vi "RMGetResults.vi"(8 "error in (no error)":errorcluster, 9 "startFrame (0)":i32, 10 "numFrames":i32, 11 "ResultManager":T4) -> (0 "error out":errorcluster, 2 "results":T1[][](array[typedef]), 3 "ResultManager (out)":T4)   [LabVIEW 2011]
uses:
  QTrkDLL.vi
  XYZf.ctl
  QTrkLocalizationJob.ctl
  QTrkLocalizationResult.ctl
  ResultManagerInstance.ctl
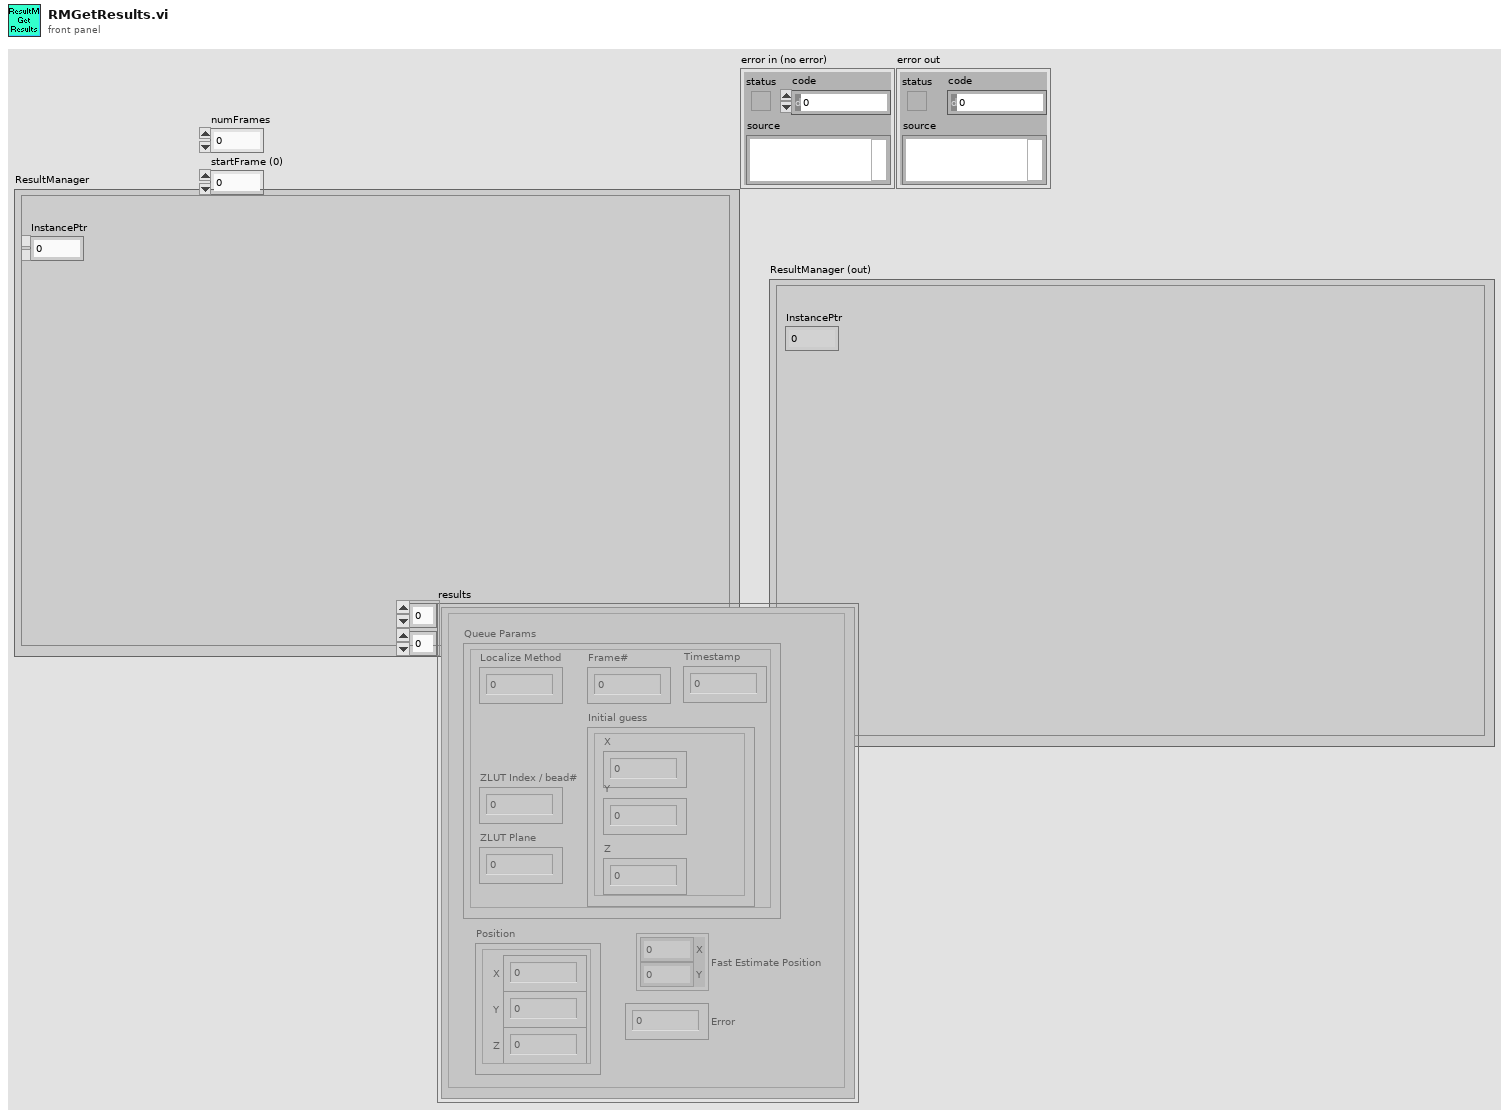
[diagram p1: front panel]
types:
  T1 = typedef "QTrkLocalizationResult.ctl" = cluster{"Queue Params":T2, "Position":T3, "Fast Estimate Position":cluster{"X":sgl, "Y":sgl}, "Error":i32}
  T2 = typedef "QTrkLocalizationJob.ctl" = cluster{"Localize Method":i32, "Frame#":u32, "Timestamp":u32, "ZLUT Index / bead#":i32, "ZLUT Plane":i32, "Initial guess":T3}
  T3 = typedef "XYZf.ctl" = cluster{"X":sgl, "Y":sgl, "Z":sgl}
  T4 = typedef "ResultManagerInstance.ctl" = cluster{"InstancePtr":u64}
  T5 = typedef "ResultManagerConfig.ctl" = cluster{"Number of beads":i32, "Number of frame info columns":i32, "Result scaling":T3, "Result offset":T3, "Write Interval":i32, "Max frames in memory":i32, "Binary output (1/0)":i8}
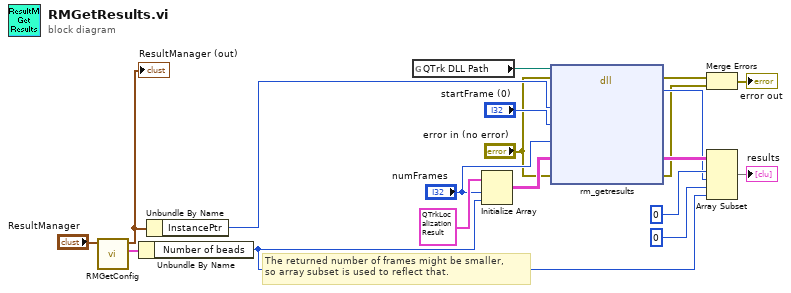
[diagram p0: block diagram]
diagram:
  # "The returned number of frames might be smaller, \nso array subset is used to reflect that."
  n1 = call "RMGetConfig.vi"("ResultManager"="ResultManager") -> ("config"=w3:T5, "ResultManager (out)"=w1:T4)  [unwired: 9 in]
  "ResultManager (out)" <- w1
  n2 = Unbundle By Name(w3) -> ("Number of beads"=w2:i32)
  n3 = Unbundle By Name(w1) -> ("InstancePtr"=w9:u64)
  n4 = global read "QTrkDLL.vi" "QTrk DLL Path"() -> (w19:path)
  n5 = Initialize Array(T1 {"Queue Params"={"Localize Method"=0, "Frame#"=0, "Timestamp"=0, "ZLUT Index / bead#"=0, "ZLUT Plane"=0, "Initial guess"={"X"=0.0, "Y"=0.0, "Z"=0.0}}, "Position"={"X"=0.0, "Y"=0.0, "Z"=0.0}, "Fast Estimate Position"={"X"=0.0, "Y"=0.0}, "Error"=0} ("Localization Result"), "numFrames", w2) -> (w17:T1[][])
  n6 = dll-call lib="D:/jcnossen1/cudaqi-tracker/bin/jtrk-labview.dll" fn="rm_getresults"(path in=w19, error in="error in (no error)", "resultmanager"=w9, "startFrame"="startFrame (0)", "numFrames"="numFrames", "results"=w17, "error"="error in (no error)") -> (error out=w7:errorcluster, "result count"=w12:i32, "results"=w14:T1[][], "error"=w6:errorcluster)  [unwired: 4 in, 1 out]
  n7 = Merge Errors(w7, w6) -> (→"error out":errorcluster)
  n8 = Array Subset(array=w14, index (row)=0 ("index"), length (row)=w12, index (col)=0 ("index"), length (col)=w2) -> (→"results":T1[][])
